vi "AlliGator Add Python Functions to Menu.vi"(8 "error in (no error)":errorcluster, 9 "Parent Menu Tag":string, 10 "Object Context Menu?":bool, 11 "Menu in":refnum<k9>) -> (0 "error out":errorcluster, 3 "Menu out":refnum<k9>)   [LabVIEW 2021, in "AlliGator Python Plugins.lvlib"]
doc: "Adds python function found in script to corresponding menu in AlliGator."
uses:
  AlliGator Python Plugins.lvlib
  AlliGator Variables List.ctl
  AlliGator Python Function Information.ctl
  AlliGator Python Function Parameter Definition.ctl
  AlliGator Python Function Output Definition.ctl
  AlliGator Python Plugin Target Type.ctl
  AlliGator Globals, Variables & Constants.lvlib
  Strings/Strings.lvlib
panel:
  # "see the AlliGator License on the block diagram (Ctrl+E or Window:Show Block Diagram)"
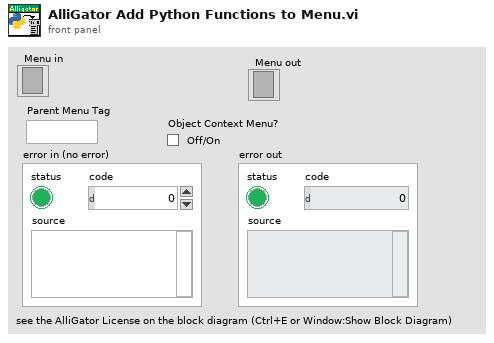
[diagram p1: front panel]
types:
  T1 = typedef "AlliGator Python Plugins.lvlib/AlliGator Python Plugin Target Type.ctl" = enum16{"Undefined", "Window Menu", "Object Menu"}
  T2 = typedef "AlliGator Python Plugins.lvlib/AlliGator Python Function Information.ctl" = cluster{"Script Path":path, "Function Name":string, "Function Parent Menu":string, "API Version":string, "Function Input Parameters":T3[], "Function Outputs":T4[], "Function Doc String":string, "Function Display Name":string, "Function Target Type":T1, "Function Target Window":string, "Parent Menu Location":string, "Item Menu Tag":string, "Is preceded by Separator":bool}
  T3 = typedef "AlliGator Python Plugins.lvlib/AlliGator Python Function Parameter Definition.ctl" = cluster{"Parameter Name":string, "Parameter Type":string, "Parameter Description":string}
  T4 = typedef "AlliGator Python Plugins.lvlib/AlliGator Python Function Output Definition.ctl" = cluster{"Output Type":string, "Output Destination":string}
  T5 = typedef "AlliGator Globals, Variables & Constants.lvlib/AlliGator Variables List.ctl" = enum16{"---- GUI ----", "GUI:Initialization Status", "GUI:State Indicators Refnum", "GUI:Original AlliGator Menu Items", "GUI:Current Action Loop State", "GUI:Script in progress", "GUI:Playback", "GUI:Loop Playback", "GUI:Search ROI Used", "GUI:Search ROI", "Decay Graph Max Legend Size", "Intensity Graph Max Legend Size", "Decay Statistics Graph Max Legend Size", "Phasor Graph Max Legend Size", "Phasor Ratio Graph Max Legend Size", "Lifetime Graph Max Legend Size", "---- Files ----", "Files:Export Dataset Frames as Individual Files", "Files:Show Batch Export Help Balloons", "Files:Frames in Dataset", "Files:ptu File Frame Start Indices", "Files:Current Frame in Dataset", "Files:Current Frame Timestamp", "Files:Dataset Loaded", "Files:Dataset Metadata", "Files:Dataset Channel", "Files:Dataset Data Description", "Files:Background Dataset Metadata", "Files:Background Dataset Channel", "Files:Background Dataset Data Description", "Files:Background File Subtraction", "Files:Background File Path", "Files:Background File Pile-up Correction", "Files:Background File Pixel Well Capacity", "Files:Background File Scaling Factor", "Files:Current Dataset Load Settings", "Files:Dataset Path", "Files:ICCD-specific Information", "Files:Macrotime Gate Separation", "------ Python Plugins ------", "Python Plugins:Information", "Python Plugins:Python Session", "Python Plugins:Valid Python Session?", "---- Source Image ----", "Source Image:ROIs", "Source Image:Current ROI", "Source Image:ROI Event Refnum", "X_Source Image Display Range", "X_Source Image Palette Information", "X_Type of Displayed Image", "X_Time Gate Slider", "Source Image:Palette List", "Source Image:Scale", "Source Image:ROI Overlay Color", "Source Image:Overlay to Erase", "Source Image:Is Displayed Image Accumulated", "Source Image:White Light Image Modified", "Source Image:Mask Image Modified", "---- Image Profile Window ----", "Image Profile:Window Event Refnum", "Image Profile:IntensityType", "Image Profile:Intensity Average Type", "Image Profile:Intensity-weighted SDV", "Image Profile:Box Profile Type", "Image Profile:Window Open", "Image Profile:Plotted Fit Parameter", "------ Phasor Graph -------", "Phasor Graph:Show Line", "---- Phasor Plot ---", "Phasor Plot:Parameters Changed", "Phasor Plot:FLI Dataset Modified since last Calculation", "Phasor Harmonics Data", "Selected Phasor Harmonics", "Phasor Harmonic Manager Event Refnum", "Phasor Plot:ROIs", "Phasor Plot:Current ROI", "Phasor Plot:ROI Event Refnum", "Phasor Plot:Image Reference Points", "Phasor Plot:Computed", "Phasor Plot:Palette Information", "Phasor Plot:Palette List", "Phasor Plot:Phasor Ratio Palette Information", "Phasor Plot:Phasor Ratio Palette List", "Phasor Plot:Image Scale", "Phasor Plot:Image Overlay to Erase", "Phasor Plot:Image Elements to Update", "Phasor Plot:Current Calculation Parameters", "Phasor Plot:Current Calibration Options", "Phasor Plot:Reset Cumulated Phasor Plot", "Phasor Plot:Reference 1", "Phasor Plot:Lifetime Reference 1", "Phasor Plot:Reference 1 Frequency", "Phasor Plot:Reference 2", "Phasor Plot:Lifetime Reference 2", "Phasor Plot:Reference 2 Frequency", "---- Decay Analysis ----", "Number of Selected Decays to Fit", "LS Fit Results", "LAR Fit Results", "BS Fit Results", "Last Decay Max - Min", "Best Fit Parameters", "Best Fit Parameter Names", "Actual Size X", "Actual Size Y", "Binning X", "Binning Y", "Actual # Gates", "Dataset Number", "Gates to...", "Gates Skipped", "Gates to keep", "Gate Step", "Gate Separation", "Reversed Gates", "Pile-up Correction", "Pixel Well Capacity", "Background Subtracted", "Background Subtraction Method", "Background Definition Range", "Background File (deprecated)", "Number of Dataset Accumulated", "Array of Accumulated Dataset Paths", "Do Averaged Datasets", "Destination File Path", "Process Plot Target", "Use 1/D as Phasor Frequency", "---- Decay Fit Parameter Map -----", "Decay Fit Parameter Map:Palette Information", "Decay Fit Parameter Map:Palette List", "------- Local Decay Window ---------", "Local Decay Graph Window:Event Refnum", "Local Decay Graph Window:Use normalized IRF for convolution", "----- Miscellaneous ----", "Misc:Skippable Dialog Windows Status"}
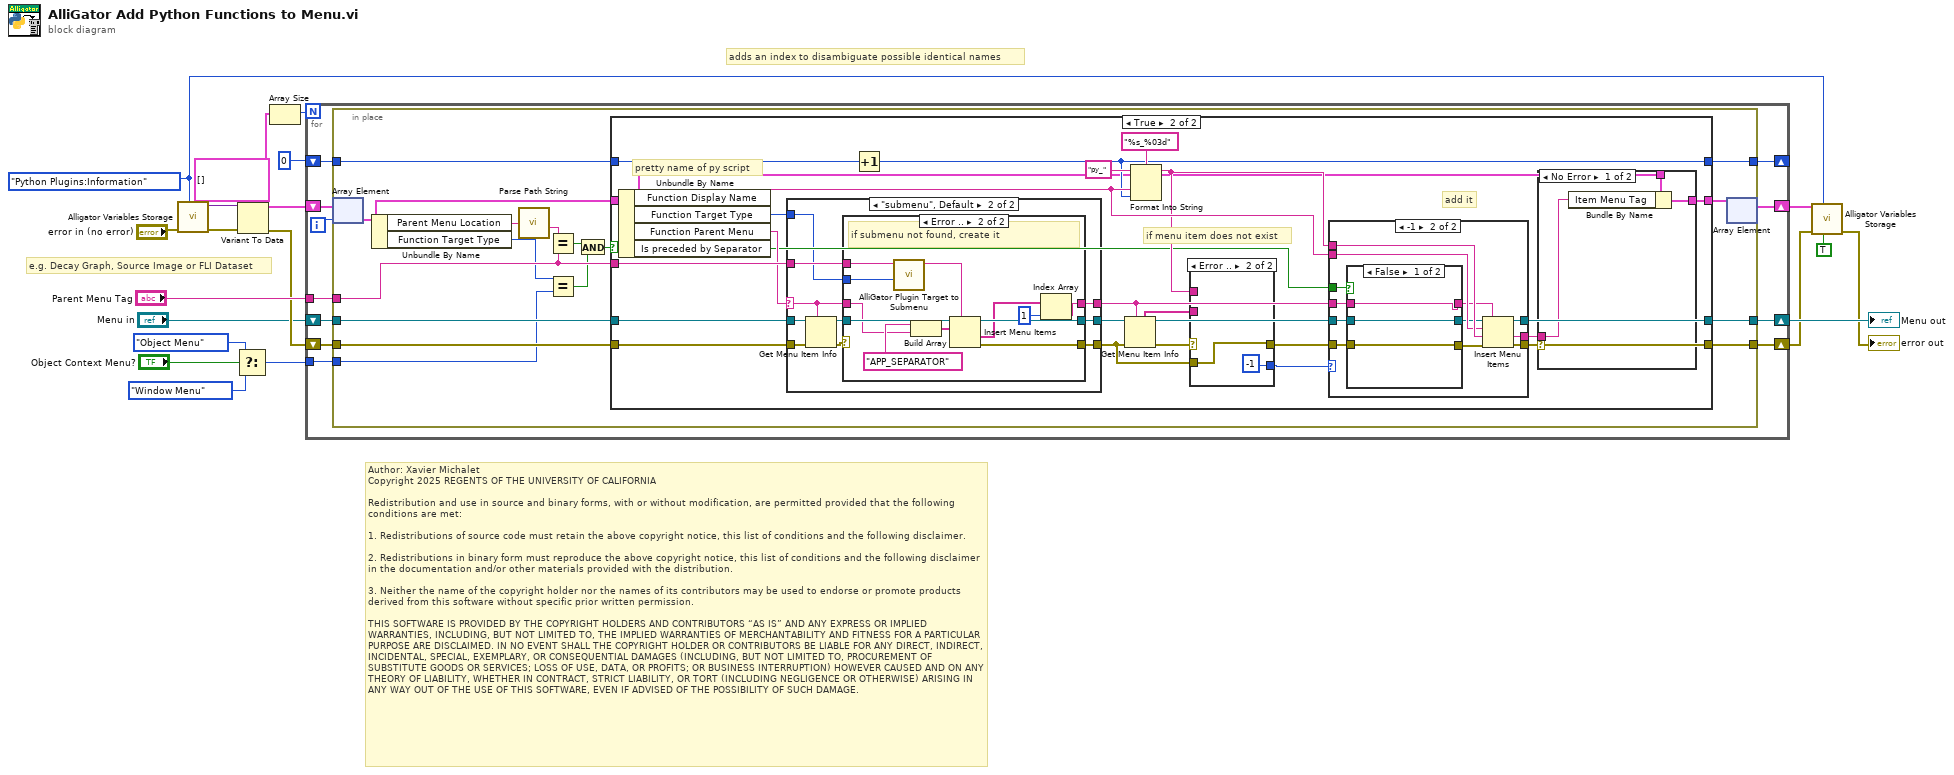
[diagram p0: block diagram]
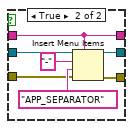
[diagram p5: hidden frame]
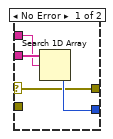
[diagram p6: hidden frame]
diagram:
  w4 = AlliGator_Variables_List."Python Plugins:Information" ("Alligator Variable")
  # "Author: Xavier Michalet\nCopyright 2025 REGENTS OF THE UNIVERSITY OF CALIFORNIA\n\nRedistribution and use in source and binary forms, with or without modification, are permitted provided that the following conditions are met:\n\n1. Redistributions of source code must retain the above copyright notice, this list of conditions and the following disclaimer.\n\n2. Redistributions in binary form must reproduce the above copyright notice, this list of conditions and the following disclaimer in the documentation and/or other materials provided with the distribution.\n\n3. Neither the name of the copyright holder nor the names of its contributors may be used to endorse or promote products derived from this software without specific prior written permission.\n\nTHIS SOFTWARE IS PROVIDED BY THE COPYRIGHT HOLDERS AND CONTRIBUTORS “AS IS” AND ANY EXPRESS OR IMPLIED WARRANTIES, INCLUDING, BUT NOT LIMITED TO, THE IMPLIED WARRANTIES OF MERCHANTABILITY AND FITNESS FOR A PARTICULAR PURPOSE ARE DISCLAIMED. IN NO EVENT SHALL THE COPYRIGHT HOLDER OR CONTRIBUTORS BE LIABLE FOR ANY DIRECT, INDIRECT, INCIDENTAL, SPECIAL, EXEMPLARY, OR CONSEQUENTIAL DAMAGES (INCLUDING, BUT NOT LIMITED TO, PROCUREMENT OF SUBSTITUTE GOODS OR SERVICES; LOSS OF USE, DATA, OR PROFITS; OR BUSINESS INTERRUPTION) HOWEVER CAUSED AND ON ANY THEORY OF LIABILITY, WHETHER IN CONTRACT, STRICT LIABILITY, OR TORT (INCLUDING NEGLIGENCE OR OTHERWISE) ARISING IN ANY WAY OUT OF THE USE OF THIS SOFTWARE, EVEN IF ADVISED OF THE POSSIBILITY OF SUCH DAMAGE."
  # "adds an index to disambiguate possible identical names"
  # "e.g. Decay Graph, Source Image or FLI Dataset"
  n1 = call "Alligator Variables Storage.vi"("AlliGator Variable"=w4, "Error In"="error in (no error)") -> ("Error Out"=w18:errorcluster, "Data out"=w19:variant)  [unwired: 7 in, 1 out]
  n2 = Select(t=AlliGator_Python_Plugin_Target_Type."Object Menu" ("Function Target Type"), s="Object Context Menu?", f=AlliGator_Python_Plugin_Target_Type."Window Menu" ("Function Target Type")) -> (s? t:f=w9:T1)
  n3 = Variant To Data(error in=w18, type=T2[] [] ("Array"), Variant=w19) -> (data=w7:T2[], error out=w16:errorcluster)
  n4 = Array Size(array=w7) -> (size(s)=w6:i32)
  n5 = for {
    N: w6 -> [_]
    tunnel: "Parent Menu Tag" -> [w27]
    shift-right: [w30] -> w14
    shift-left: "Menu in" -> [w31]
    shift-right: [w28] -> w3
    shift-left: w16 -> [w29]
    tunnel: w9 -> [w26]
    shift-right: [w24] -> _
    shift-left: 0 ("input 2") -> [w25]
    shift-right: [w22] -> w5
    shift-left: w7 -> [w23]
    i -> [w21]
    n6 = in-place {
      in-place-border: w31 -> [w47]
      in-place-border: [w46] -> w30
      in-place-border: w29 -> [w45]
      in-place-border: [w44] -> w28
      in-place-border: w27 -> [w43]
      in-place-border: w26 -> [w39]
      in-place-border: w25 -> [w35]
      in-place-border: [w34] -> w24
      n7 = in-place-array #1(w23, w21) -> (w33:T2)
      n8 = Unbundle By Name(w33) -> ("Parent Menu Location"=w42:string, "Function Target Type"=w40:T1)
      n9 = call "Parse Path String.vi"("Path in"=w42) -> ("File/Folder"=w41:string)  [unwired: 4 in, 1 out]
      n10 = Equal?(x=w41, y=w43) -> (x = y?=w38:bool)
      n11 = Equal?(x=w40, y=w39) -> (x = y?=w37:bool)
      n12 = And(x=w38, y=w37) -> (x .and. y?=w36:bool)
      n13 = case shown="True" w36 {
        tunnel: w47 -> [w51 w76]
        tunnel: [w51 w75] -> w46
        tunnel: w45 -> [w50 w74]
        tunnel: [w50 w55] -> w44
        tunnel: w43 -> [_ w73]
        tunnel: w33 -> [w48 w58]
        tunnel: w35 -> [w49 w60]
        tunnel: [w49 w59] -> w34
        tunnel: [w48 w56] -> w32
        frame False {
        }
        frame True {
          # "add it"
          # "if menu item does not exist"
          # "pretty name of py script"
          n14 = Unbundle By Name(w58) -> ("Function Display Name"=w62:string, "Function Target Type"=w65:T1, "Function Parent Menu"=w66:string, "Is preceded by Separator"=w54:bool)
          n15 = case shown="\"submenu\", Default" w66 {
            selector: w66 -> [_ w118]
            tunnel: w76 -> [w112 w122]
            tunnel: w74 -> [w111 w121]
            tunnel: [w112 w117] -> w72
            tunnel: [w111 w116] -> w52
            tunnel: [_ w115] -> w70
            tunnel: w73 -> [_ w114]
            tunnel: w65 -> [_ w113]
            frame "" {
            }
            frame "submenu", Default {
              n16 = Get Menu Item Info(7:w118, 8:w121, 11:w122) -> (0:w120:errorcluster, 3:w119:refnum<k9>)  [unwired: 5 out]
              n17 = case shown="Error .." w120 {
                selector: w120 -> [w124 _]
                tunnel: w119 -> [w125 w137]
                tunnel: w118 -> [w123 w127]
                tunnel: [w125 w136] -> w117
                tunnel: [w124 w135] -> w116
                tunnel: [w123 w131] -> w115
                tunnel: w114 -> [_ w129]
                tunnel: w113 -> [_ w126]
                frame No Error {
                }
                frame Error {
                  # "if submenu not found, create it"
                  n18 = call "AlliGator Plugin Target to Submenu.vi"("Function Target Type"=w126, "Function Target"=w129) -> ("Menu Tag"=w128:string)  [unwired: 9 in]
                  n19 = Build Array("APP_SEPARATOR" ("element"), w127) -> (w133:string[])
                  n20 = Insert Menu Items(5:w128, 8:w133, 9:w137) -> (0:w135:errorcluster, 1:w134:string[], 3:w136:refnum<k9>)  [unwired: 3 in]
                  n21 = Index Array(array=w134, index=1) -> (element=w131:string)
                }
              }
            }
          }
          n22 = Increment(x=w60) -> (x+1=w59:i32)
          n23 = Get Menu Item Info(7:w70, 8:w52, 11:w72) -> (0:w69:errorcluster, 3:w71:refnum<k9>, 5:w68:string[])  [unwired: 4 out]
          n24 = Format Into String(format string="%s_%03d", initial string="py_" ("string"), w62, w59) -> (resulting string=w61:string)  [unwired: 1 in, 1 out]
          n25 = case shown="Error .." w69 {
            selector: w69 -> [w105 _]
            tunnel: w68 -> [w108 _]
            tunnel: w61 -> [w107 _]
            tunnel: [w106 -1 ("index of element")] -> w67
            tunnel: [w105 w109] -> w53
            tunnel: w52 -> [_ w109]
            frame No Error {
              n26 = Search 1D Array(1D array=w108, element=w107) -> (index of element=w106:i32)  [unwired: 1 in]
            }
            frame Error {
            }
          }
          n27 = case shown="-1" w67 {
            tunnel: [w82 w94] -> w75
            tunnel: [_ w93] -> w55
            tunnel: w61 -> [w81 w92]
            tunnel: w71 -> [w82 w88]
            tunnel: w70 -> [_ w86]
            tunnel: w62 -> [_ w91]
            tunnel: [w81 w90] -> w57
            tunnel: w54 -> [_ w89]
            tunnel: w53 -> [_ w84]
            frame 0, Default {
            }
            frame -1 {
              n28 = case shown="False" w89 {
                tunnel: w88 -> [w97 w104]
                tunnel: [w97 w103] -> w87
                tunnel: w86 -> [w95 w98]
                tunnel: [w96 w100] -> w85
                tunnel: w84 -> [w96 w99]
                tunnel: [w95 w98] -> w83
                frame False {
                }
                frame True {
                  n29 = Insert Menu Items(5:w98, 6:w99, 7:"APP_SEPARATOR" ("item tags"), 8:"-" ("item names"), 9:w104) -> (0:w100:errorcluster, 3:w103:refnum<k9>)  [unwired: 1 in, 1 out]
                }
              }
              n30 = Insert Menu Items(5:w83, 6:w85, 7:w92, 8:w91, 9:w87) -> (0:w93:errorcluster, 1:w90:string, 3:w94:refnum<k9>)  [unwired: 1 in]
            }
          }
          n31 = case shown="No Error" w55 {
            tunnel: w58 -> [w79 w80]
            tunnel: w57 -> [w78 _]
            tunnel: [w77 w80] -> w56
            frame No Error {
              n32 = Bundle By Name(cluster=w79, "Item Menu Tag"=w78) -> (w77:T2)
            }
            frame Error {
            }
          }
        }
      }
      n33 = in-place-array #1(w32) -> (w22:T2[])  [unwired: 1 out]
    }
  }
  "Menu out" <- w14
  n34 = call "Alligator Variables Storage.vi"("Get(F)/Set"=TRUE, "AlliGator Variable"=w4, "Error In"=w3, "Data in"=w5) -> ("Error Out"=→"error out":errorcluster)  [unwired: 5 in, 2 out]
